vi "GPS Handler.vi"() -> ()   [LabVIEW 2023]
uses:
  <vilib>/LabVIEW Targets/FPGA/cRIO/shared/nicrio_ModuleControls/nicrio_cRIO-9467_Latitude.ctl
  <vilib>/LabVIEW Targets/FPGA/cRIO/shared/nicrio_ModuleControls/nicrio_cRIO-9467_Longitude.ctl
  <vilib>/LabVIEW Targets/FPGA/cRIO/shared/nicrio_ModuleControls/nicrio_cRIO-9467_Altitude.ctl
  <vilib>/rvi/Emulation/niFpgaGetClockAttributes.vi
  <vilib>/rvi/Emulation/niFpgaSctlEmulationGetInTimedLoop.vi
  <vilib>/rvi/Emulation/niFpgaEmulationReportErrorSimple.vi
  <vilib>/rvi/eio/common/nirviEmuTemplateMethod_errors.vi
  <vilib>/rvi/eio/common/nirviEmuTemplatePropertyGet_errors.vi
  <vilib>/rvi/Emulation/niFpgaCriticalErrorInLSC.vi
  <vilib>/eio/EIOMethodNode/EIOMethodNode.xnode
  <vilib>/eio/EIOPropertyNode/EIOPropertyNode.xnode
  <vilib>/rvi/eio/common/nirviEmuTemplatePropertyGet_noerrors.vi
  <vilib>/rvi/eio/common/nirviEmuTemplatePropertySet_errors.vi
  <vilib>/rvi/eio/common/nirviEmuTemplatePropertySet_noerrors.vi
panel:
  out "Vendor ID":u16
  out "UTC Offset Valid":bool
  out "UTC Offset":i8
  out "Serial Number":u32
  out "Module ID":u16
  out "Leap Second Pending":bool
  out "Leap Second Occurred":bool
  out "Leap Second Direction":enum8{"Add", "Delete"}(ring)
  out "GPS Status":T1(ring)
  out "Firmware Version":u32
  out "Antenna Status":T2(ring)
  out "Self-Survey Complete":bool
  out "Satellites Available":u8
  out "PPS Timestamp (TAI)":u64
  out "Altitude (m)":T3 format="%.2f"
  out "Longitude (°)":T4 format="%.6g"
  out "Latitude (°)":T5 format="%.6f"
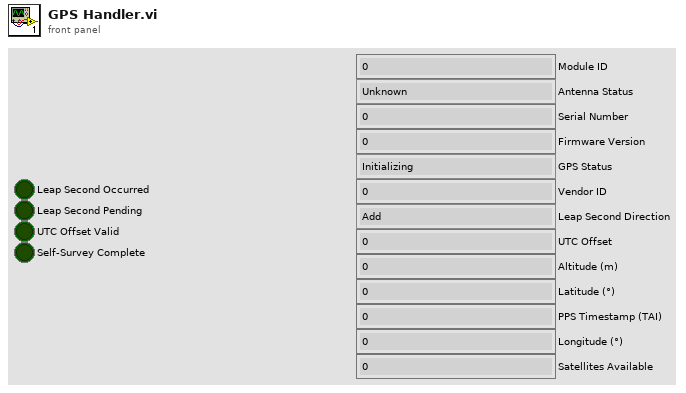
[diagram p1: front panel]
types:
  T1 = enum8{"Initializing", "Normal", "Unable to get fix"}
  T2 = enum8{"Unknown", "Normal", "Absent", "Overcurrent"}
  T3 = typedef "nicrio_cRIO-9467_Altitude.ctl" = fxp<+/-,24,17>
  T4 = typedef "nicrio_cRIO-9467_Longitude.ctl" = fxp<+/-,29,9>
  T5 = typedef "nicrio_cRIO-9467_Latitude.ctl" = fxp<+/-,28,8>
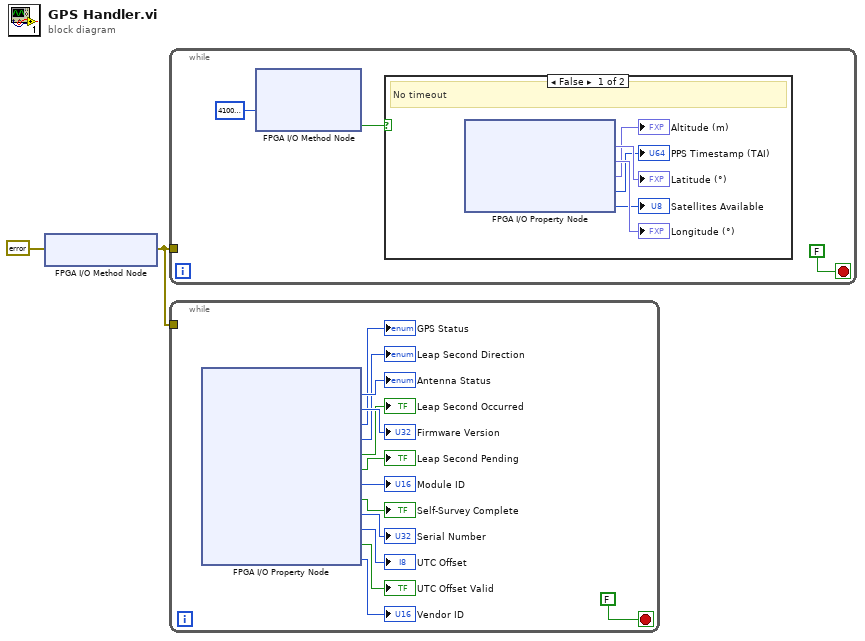
[diagram p0: block diagram]
diagram:
  n1 = xnode "FPGA I/O Method Node"("error in"=errorcluster {"status"=FALSE, "code"=0, "source"=""} ("error out")) -> ("error out"=w1:errorcluster)  [unwired: 1 in, 1 out]
  n2 = while {
    tunnel: w1 -> [_]
    stop <- FALSE stop-if-true
    n3 = xnode "FPGA I/O Method Node"("Timeout"=41000000) -> ("Timed Out"=w3:bool)  [unwired: 2 in, 2 out]
    n4 = case shown="False" w3 {
      frame False {
        # "No timeout"
        n5 = xnode "FPGA I/O Property Node"() -> ("Latitude (°)"=→"Latitude (°)":T5, "Longitude (°)"=→"Longitude (°)":T4, "Altitude (m)"=→"Altitude (m)":T3, "PPS Timestamp (TAI)"=→"PPS Timestamp (TAI)":u64, "Satellites Available"=→"Satellites Available":u8)  [unwired: 2 in, 2 out]
      }
      frame True {
        # "Timeout"
      }
    }
  }
  n6 = while {
    tunnel: w1 -> [_]
    stop <- FALSE stop-if-true
    n7 = xnode "FPGA I/O Property Node"() -> ("Antenna Status"=→"Antenna Status":T2, "Firmware Version"=→"Firmware Version":u32, "GPS Status"=→"GPS Status":T1, "Leap Second Direction"=→"Leap Second Direction":enum8{"Add", "Delete"}, "Leap Second Occurred"=→"Leap Second Occurred":bool, "Leap Second Pending"=→"Leap Second Pending":bool, "Module ID"=→"Module ID":u16, "Self-Survey Complete"=→"Self-Survey Complete":bool, "Serial Number"=→"Serial Number":u32, "UTC Offset"=→"UTC Offset":i8, "UTC Offset Valid"=→"UTC Offset Valid":bool, "Vendor ID"=→"Vendor ID":u16)  [unwired: 2 in, 2 out]
  }
